vi "ReadConfig.vi"(0 "reference in":refnum<class "Sig_Digital.lvclass">, 11 "error in (no error)":errorcluster) -> (4 "reference out":refnum<class "Sig_Digital.lvclass">, 15 "error out":errorcluster)   [LabVIEW 2019, in "Sig_Digital.lvclass"]
uses:
  Sig_Digital.lvclass
  D:/GIT H4000/H4000/src/Proccess_class/Proccess.lvclass
  Sig_Digital.lvclass/Sig_Digital.ctl
  Proccess_class/Proccess.lvclass/Proccess.ctl
  164634c0-10a3-4ec1-8939-5c81fd15110d.vi
  <vilib>/Utility/error.llb/Clear Errors.vi
  ConfigInterface_class/ConfigInterface.lvclass
  Proccess_class/Proccess.lvclass
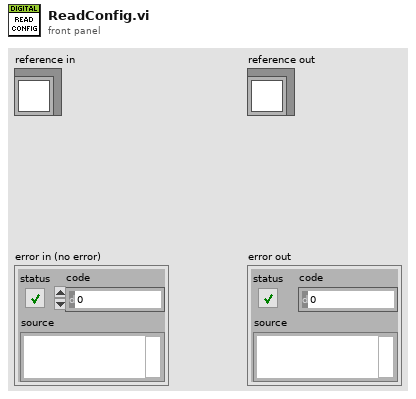
[diagram p1: front panel]
types:
  T1 = typedef "Config_Digital.ctl" = cluster{"Invert":bool, "AlarmEnable":bool, "AlarmValueEU":bool, "WarningEnable":bool, "WarningValueEU":bool, "AlarmTime":dbl}
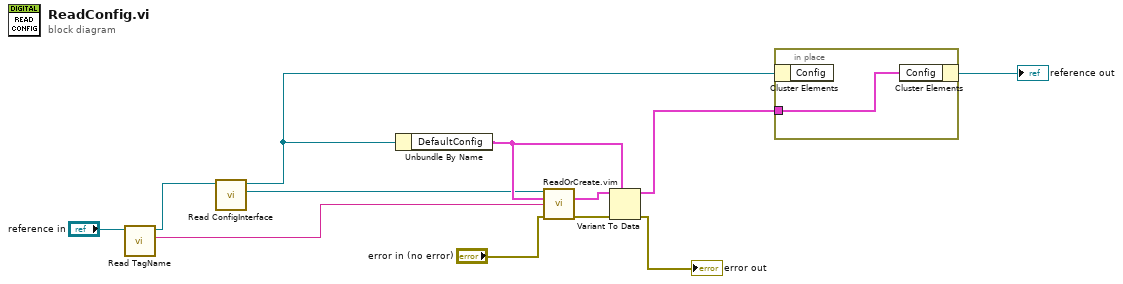
[diagram p0: block diagram]
diagram:
  n1 = call "Read TagName.vi"("Proccess in"="reference in") -> ("TagName"=w6:string, "Proccess out"=w2:refnum<class "Sig_Digital.lvclass">)  [unwired: 9 in]
  n2 = call "Read ConfigInterface.vi"("Proccess in"=w2) -> ("ConfigInterface"=w5:refnum<class "ConfigInterface.lvclass">, "Proccess out"=w1:refnum<class "Sig_Digital.lvclass">)  [unwired: 9 in]
  n3 = Unbundle By Name(w1) -> ("DefaultConfig"=w7:T1)
  n4 = call "ReadOrCreate.vim"("reference in"=w5, "Type and Defaults"=w7, "Name"=w6, "error in (no error)"="error in (no error)") -> ("Data"=w9:T1, "error out"=w10:errorcluster)  [unwired: 7 in, 3 out]
  n5 = Variant To Data(error in=w10, type=w7, Variant=w9) -> (data=w11:T1, error out=→"error out":errorcluster)
  n6 = in-place {
    in-place-border: w11 -> [w13]
    n7 = in-place-cluster #1(w1) -> ()  [unwired: 1 out]
    n8 = in-place-cluster #1("Config"=w13) -> (→"reference out":refnum<class "Sig_Digital.lvclass">)
  }
